vi "TCP create listener.vi"(7 "net address":u32, 8 "error in (no error)":errorcluster, 9 "timeout ms (25000)":i32=25000, 10 "port":u16, 11 "service name":string) -> (0 "error out":errorcluster, 2 "port out":u16, 3 "TCP out":refnum<class "TCP.lvclass">)   [LabVIEW 2013, in "TCP.lvclass"]
doc: "Creates a listener for a TCP network connection. Wire 0 to the port input to dynamically choose an available TCP port the operating system determines is valid for use. Use the TCP Open Connection to query the NI Service Locator for the port number registered with the service name"
uses:
  TCP.lvclass
  TCP.lvclass/TCP.ctl
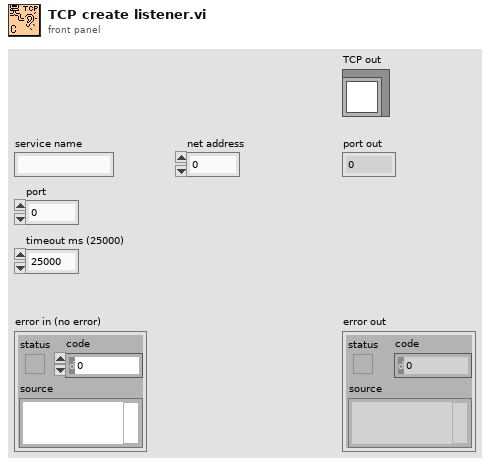
[diagram p1: front panel]
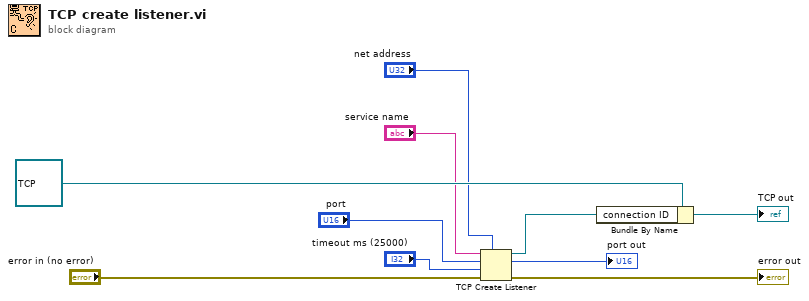
[diagram p0: block diagram]
diagram:
  n1 = TCP Create Listener(7:"net address", 8:"error in (no error)", 9:"timeout ms (25000)", 10:"port", 11:"service name") -> (0:→"error out":errorcluster, 2:→"port out":u16, 3:w1:refnum<k5>)
  n2 = Bundle By Name(cluster=refnum<class "TCP.lvclass"> refnum ("TCP in"), "connection ID"=w1) -> (→"TCP out":refnum<class "TCP.lvclass">)
